vi "other labview thingy.vi"() -> ()   [LabVIEW 2020]
panel:
  in  "stop":bool
  out "Thermometer":dbl(slide) scale=0.0..100.0
  out "element 2":string
  out "element":string
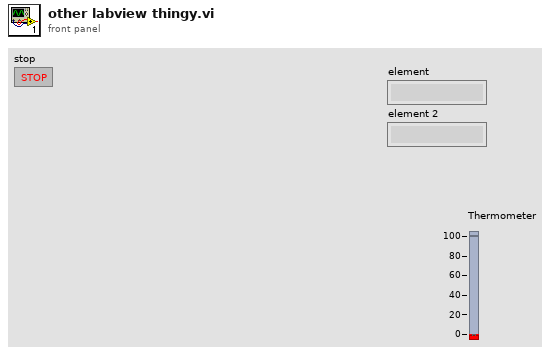
[diagram p1: front panel]
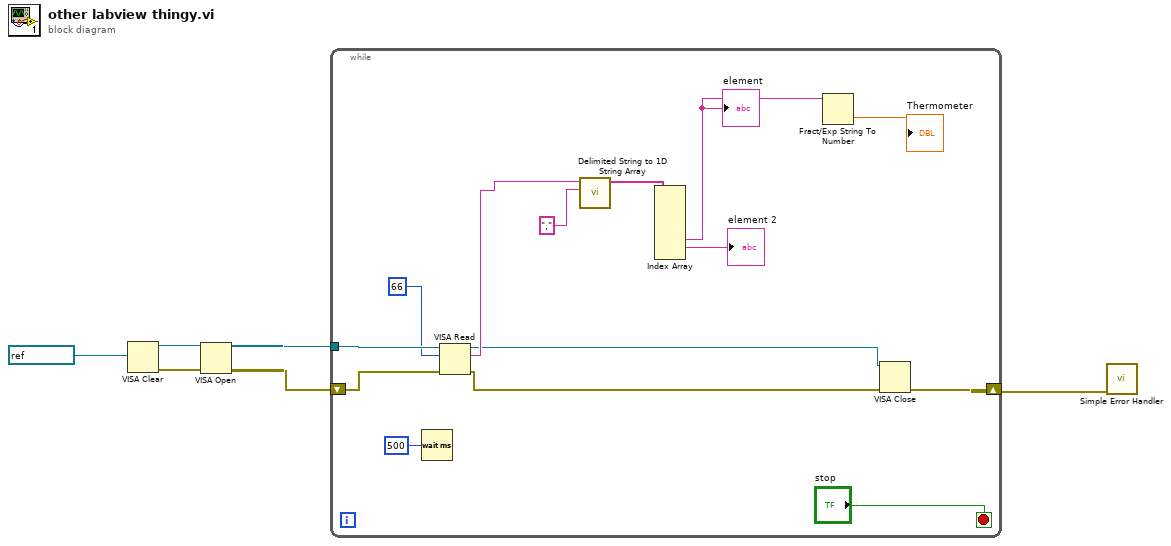
[diagram p0: block diagram]
diagram:
  n1 = VISA Clear(VISA resource name=refnum<visa-resource-name> "COM13") -> (VISA resource name out=w6:refnum<visa-resource-name>, error out=w5:errorcluster)  [unwired: 1 in]
  n2 = VISA Open(error in (no error)=w5, VISA resource name=w6) -> (VISA resource name=w4:refnum<visa-resource-name>, error out=w3:errorcluster)  [unwired: 3 in]
  n3 = while {
    tunnel: w4 -> [w20]
    shift-right: [w11] -> w2
    shift-left: w3 -> [w19]
    stop <- "stop" stop-if-true
    n4 = Wait (ms)(milliseconds to wait=u32 500) -> ()  [unwired: 1 out]
    n5 = VISA Read(VISA resource name=w20, byte count=u32 66, error in (no error)=w19) -> (VISA resource name out=w12:refnum<visa-resource-name>, read buffer=w17:string, error out=w13:errorcluster)  [unwired: 1 out]
    n6 = call <vilib>:"Delimited String to 1D String Array.vi"("delimiter"=",", "delimited string"=w17) -> ("string array"=w15:string[])  [unwired: 9 in]
    n7 = Index Array(array=w15) -> (element #5=w9:string, element #6=→"element 2":string)  [unwired: 7 in, 5 out]
    "element" <- w9
    n8 = Fract/Exp String To Number(string=w9) -> (number=→"Thermometer":dbl)  [unwired: 3 in, 1 out]
    n9 = VISA Close(VISA resource name=w12, error in (no error)=w13) -> (error out=w11:errorcluster)
  }
  n10 = call <vilib>:"Simple Error Handler.vi"("error in (no error)"=w2) -> ()  [unwired: 4 in, 5 out]
